vi "CheckListener ConvBox Handler.vi"(8 "error in (no error)":errorcluster, 11 "Listener in":refnum<class "Listener.lvclass">) -> (0 "error out":errorcluster, 3 "Listener out":refnum<class "Listener.lvclass">)   [LabVIEW 2023, in "Listener.lvclass"]
uses:
  Listener.lvclass
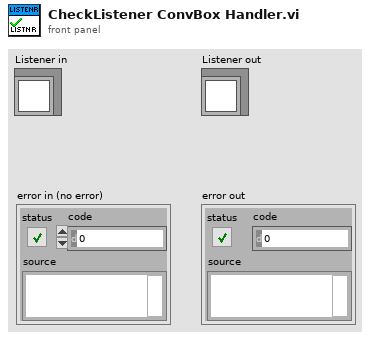
[diagram p1: front panel]
types:
  T1 = typedef "Listener.lvclass/RS-xxx To GPIB ConvBox Data Structure.ctl" = cluster{"Data":string, "Command Messages Read":string[], "Address":string, "Data Length":u32}
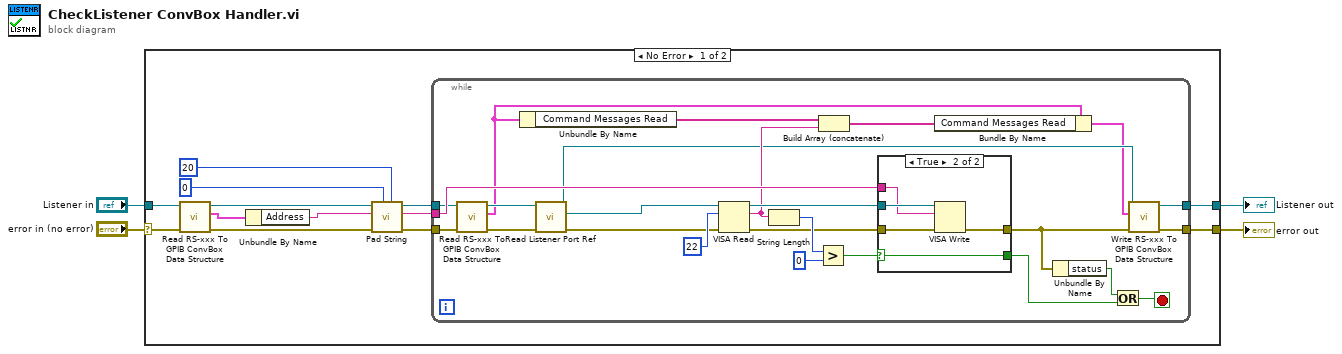
[diagram p0: block diagram]
diagram:
  n1 = case shown="No Error" "error in (no error)" {
    selector: "error in (no error)" -> [w14 w51]
    tunnel: [w17 w51] -> w4
    tunnel: "Listener in" -> [w15 w50]
    tunnel: [w16 w50] -> w1
    frame No Error {
      n2 = call-dynamic "Read RS-xxx To GPIB ConvBox Data Structure.vi"("error in (no error)"=w14, "Listener in"=w15) -> ("error out"=w12:errorcluster, "RS-xxx To GPIB ConvBox Data Structure"=w13:T1, "Listener out"=w9:refnum<class "Listener.lvclass">)  [unwired: 7 in]
      n3 = Unbundle By Name(w13) -> ("Address"=w10:string)
      n4 = call "Pad String.vi"("Expected Length"=u8 20, "Pad Character"=u8 0, "error in (no error)"=w12, "String To Pad"=w10, "Listener in"=w9) -> ("error out"=w11:errorcluster, "Padded String"=w6:string, "Listener out"=w5:refnum<class "Listener.lvclass">)  [unwired: 4 in]
      n5 = while {
        tunnel: w6 -> [w33]
        tunnel: w11 -> [w30]
        tunnel: [w23] -> w17
        tunnel: w5 -> [w31]
        tunnel: [w22] -> w16
        stop <- w37 stop-if-true
        n6 = call-dynamic "Read RS-xxx To GPIB ConvBox Data Structure.vi"("error in (no error)"=w30, "Listener in"=w31) -> ("error out"=w29:errorcluster, "RS-xxx To GPIB ConvBox Data Structure"=w20:T1, "Listener out"=w27:refnum<class "Listener.lvclass">)  [unwired: 7 in]
        n7 = Unbundle By Name(w20) -> ("Command Messages Read"=w26:string[])
        n8 = call "Read Listener Port Ref.vi"("error in (no error)"=w29, "Listener in"=w27) -> ("error out"=w28:errorcluster, "Listener Port Ref"=w32:refnum<visa-resource-name>, "Listener out"=w21:refnum<class "Listener.lvclass">)  [unwired: 7 in]
        n9 = VISA Read(VISA resource name=w32, byte count=u32 22, error in (no error)=w28) -> (VISA resource name out=w41:refnum<visa-resource-name>, read buffer=w25:string, error out=w34:errorcluster)  [unwired: 1 out]
        n10 = String Length(string=w25) -> (length=w40:i32)
        n11 = Greater?(x=w40, y=0) -> (0:w38:bool)
        n12 = Build Array (concatenate)(w26, w25) -> (w19:string[])
        n13 = case shown="True" w38 {
          selector: w38 -> [w44 w47]
          tunnel: w34 -> [w43 w49]
          tunnel: w41 -> [_ w48]
          tunnel: [w44 w47] -> w36
          tunnel: [w43 w46] -> w24
          tunnel: w33 -> [_ w45]
          frame False {
          }
          frame True {
            n14 = VISA Write(VISA resource name=w48, write buffer=w45, error in (no error)=w49) -> (error out=w46:errorcluster)  [unwired: 2 out]
          }
        }
        n15 = Bundle By Name(cluster=w20, "Command Messages Read"=w19) -> (w18:T1)
        n16 = Unbundle By Name(w24) -> ("status"=w35:bool)
        n17 = Or(x=w35, y=w36) -> (x .or. y?=w37:bool)
        n18 = call-dynamic "Write RS-xxx To GPIB ConvBox Data Structure.vi"("error in (no error)"=w24, "RS-xxx To GPIB ConvBox Data Structure"=w18, "Listener in"=w21) -> ("error out"=w23:errorcluster, "Listener out"=w22:refnum<class "Listener.lvclass">)  [unwired: 7 in]
      }
    }
    frame Error {
    }
  }
  "error out" <- w4
  "Listener out" <- w1
